vi "LS340_ConfigChannel.vi"(0 "VISA resource name":refnum<visa-resource-name>, 1 "Configure (F:Don't Config)":bool, 2 "Delay After Config (1000 ms)":u32=1000 min=1000 max=99999 step=1, 3 "Manual Output (0.00)":dbl min=0.0 max=100.0 step=0.01 format="%.2f", 5 "Loop (0: 1)":u16(ring) items=["1", "2"], 7 "Gain (P) (0.0)":dbl min=0.0 max=1000.0 step=0.1 format="%.1f", 9 "Reset (I) (0.0)":dbl min=0.0 max=1000.0 step=0.1 format="%.1f", 11 "error in (no error)":errorcluster, 12 "Rate (D) (0)":dbl min=0.0 max=1000.0 step=1.0, 13 "Heater Range (0: Off)":u16(ring) items=["Off", "1", "2", "3", "4", "5"], 14 "Setpoint (0.0)":dbl min=-273.0 max=300000.0 step=0.0001 format="%.4f") -> (4 "VISA out":refnum<visa-resource-name>, 15 "error out":errorcluster)   [LabVIEW 2012]
doc: "This VI was designed to demonstrate typical usage of sub vi's containing the more common 340 functions.\n\nThis example configures the loop and setpoint of the instrument, allows for a delay, and then reads sensor and heater output data. The user is given the option of just reading data and not configuring the instrument."
uses:
  <instrlib>/Lake Shore Cryotronics 340/Lake Shore Cryotronics 340.lvlib
panel:
  # "Copyright 2005. National Instruments Corporation"
  # "Configure\nDo Not Configure"
  # "340 Temperature Controller"
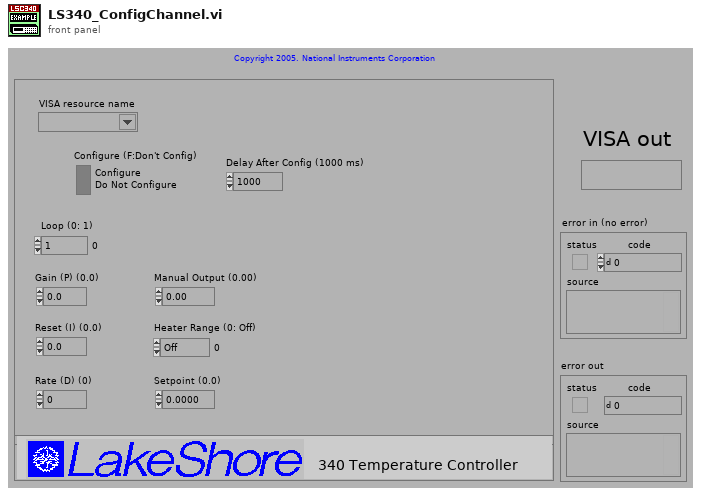
[diagram p1: front panel]
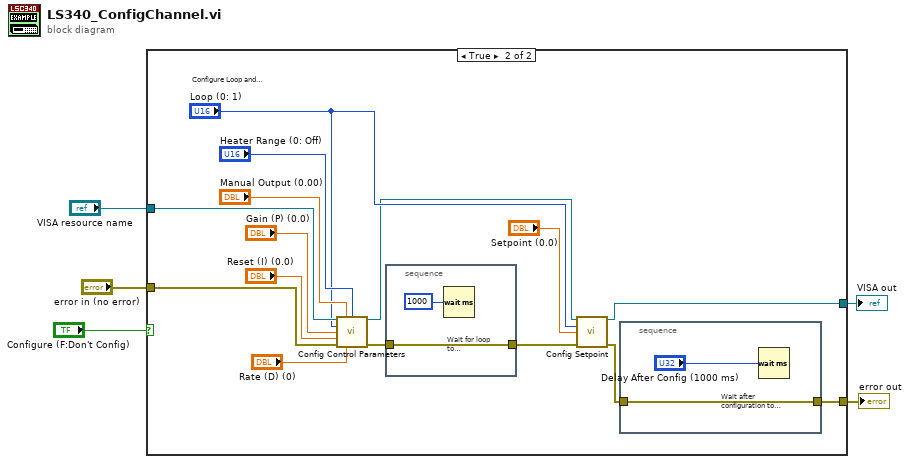
[diagram p0: block diagram]
diagram:
  n1 = case shown="True" "Configure (F:Don't Config)" {
    tunnel: "error in (no error)" -> [w6 w22]
    tunnel: "VISA resource name" -> [w7 w18]
    tunnel: [w6 w9] -> w2
    tunnel: [w7 w8] -> w1
    frame False {
      # "Do not configure Loop and Setpoint."
    }
    frame True {
      # "Configure Loop and Setpoint."
      n2 = call <instrlib>:"Config Control Parameters.vi"("VISA resource name"=w18, "Manual Output (0.00)"="Manual Output (0.00)", "Heater Range (0: Off)"="Heater Range (0: Off)", "Loop (0: 1)"="Loop (0: 1)", "Gain (P) (0.0)"="Gain (P) (0.0)", "Reset (I) (0.0)"="Reset (I) (0.0)", "error in (no error)"=w22, "Rate (D) (0)"="Rate (D) (0)") -> ("VISA resource name out"=w12:refnum<visa-resource-name>, "error out"=w15:errorcluster)  [unwired: 6 in]
      n3 = stacked-sequence {
        tunnel: w15 -> [w25]
        tunnel: [w25] -> w14
        frame #0 {
          # "Wait for loop to \nconfigure."
          n4 = Wait (ms)(milliseconds to wait=u32 1000) -> ()  [unwired: 1 out]
        }
      }
      n5 = call <instrlib>:"Config Setpoint.vi"("VISA resource name"=w12, "Loop (0: 1)"="Loop (0: 1)", "Setpoint (0.0)"="Setpoint (0.0)", "error in (no error)"=w14) -> ("VISA resource name out"=w8:refnum<visa-resource-name>, "error out"=w10:errorcluster)  [unwired: 10 in]
      n6 = stacked-sequence {
        tunnel: w10 -> [w24]
        tunnel: [w24] -> w9
        frame #0 {
          # "Wait after configuration to\nread data."
          n7 = Wait (ms)(milliseconds to wait="Delay After Config (1000 ms)") -> ()  [unwired: 1 out]
        }
      }
    }
  }
  "error out" <- w2
  "VISA out" <- w1
